vi "试剂余量百分比确认.vi"(11 "试剂余量百分比 2":u16 caption="试剂容量") -> (3 "Value":u16, 5 "check ？":bool)   [LabVIEW 2016, in "斯坦道通用流路CODmn.lvlib"]
panel:
  in  "确认":bool
  in  "关闭":bool
  in  "试剂余量百分比":u16=100 format="%.0f %%"
  # "请输入试剂余量百分比"
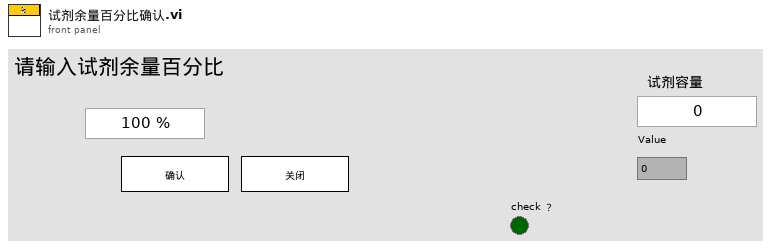
[diagram p1: front panel]
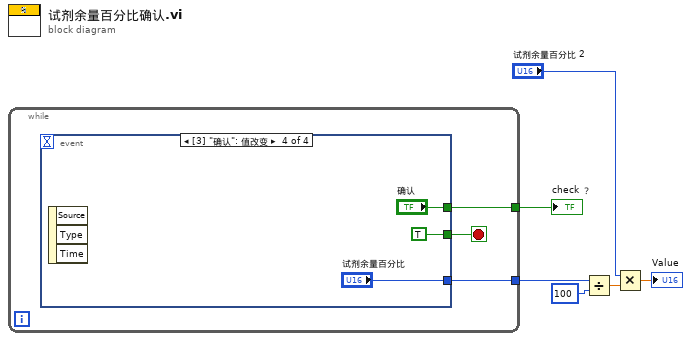
[diagram p0: block diagram]
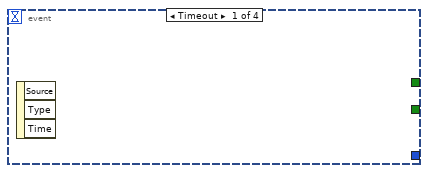
[diagram p2: hidden frame]
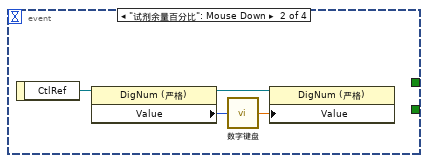
[diagram p3: hidden frame]
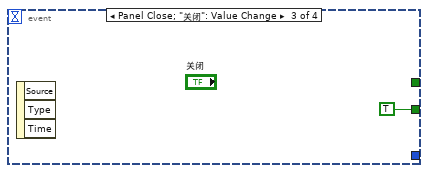
[diagram p4: hidden frame]
diagram:
  n1 = while {
    tunnel: [w8] -> w6
    tunnel: [w7] -> w1
    stop <- w9 stop-if-true
    n2 = event shown="[3] \"确认\": 值改变" {
      selector: _ -> [_ _ _ _]
      dyn-events: _ -> [_ _ _ _]
      timeout: _ -> [_ _ _ _]
      tunnel: [_ _ TRUE TRUE] -> w9
      tunnel: [_ _ _ "试剂余量百分比"] -> w8
      tunnel: [_ _ _ "确认"] -> w7
      event Timeout {
        n3 = event-data() -> ()  [unwired: 1 in, 3 out]
      }
      event "试剂余量百分比": Mouse Down {
        n4 = event-data() -> ("CtlRef"=w13:refnum<vi>)  [unwired: 1 in]
        n5 = property class="DigNum (严格)"(reference=w13) -> (reference out=w10:refnum<vi>, "Value"=w12:u16)  [unwired: 1 in, 1 out]
        n6 = call "数字键盘.vi"("OldNumber"=w12) -> ("NewNumber"=w11:dbl)
        n7 = property class="DigNum (严格)"(reference=w10, "Value"=w11) -> ()  [unwired: 1 in, 2 out]
      }
      event Panel Close; "关闭": Value Change {
        n8 = event-data() -> ()  [unwired: 1 in, 3 out]
      }
      event "确认": Value Change {
        n9 = event-data() -> ()  [unwired: 1 in, 3 out]
      }
    }
  }
  "check ？" <- w1
  n10 = Divide(x=w6, y=u16 100) -> (x/y=w4:dbl)
  n11 = Multiply(x="试剂余量百分比 2", y=w4) -> (x*y=→"Value":dbl)
